vi "UpdateValve.vi"(8 "error in (no error)":errorcluster, 11 "Pump_1AI_1DO_2DI in":refnum<class "Valve_2DO_2DI.lvclass">) -> (0 "error out":errorcluster, 3 "Pump_1AI_1DO_2DI out":refnum<class "Valve_2DO_2DI.lvclass">)   [LabVIEW 2019, in "Valve_2DO_2DI.lvclass"]
uses:
  Valve_2DO_2DI.lvclass
  C:/Users/H4001/Documents/GitHub/H4000/src/Device_class/Device.lvclass
  Device_class/Device.lvclass/Device.ctl
  Valve_2DO_2DI.lvclass/Valve_2DO_2DI.ctl
  DA_class/DA.lvclass/DA.ctl
  Proccess_class/Proccess.lvclass/Proccess.ctl
  FPGA/TypeDef/valveState.ctl
  subvis/bool_change.vi
  DA_class/private/write_to_db.vi
  Proccess_class/GetNames.vi
  Proccess_class/GetLogger.vi
  DA_class/DA.lvclass
  C:/Users/H4001/Documents/GitHub/H4000/src/Proccess_class/Proccess.lvclass
  Logger_class/WriteEvent.vi
  FPGA_API_class/FPGA API.lvclass
  Device_class/Device.lvclass
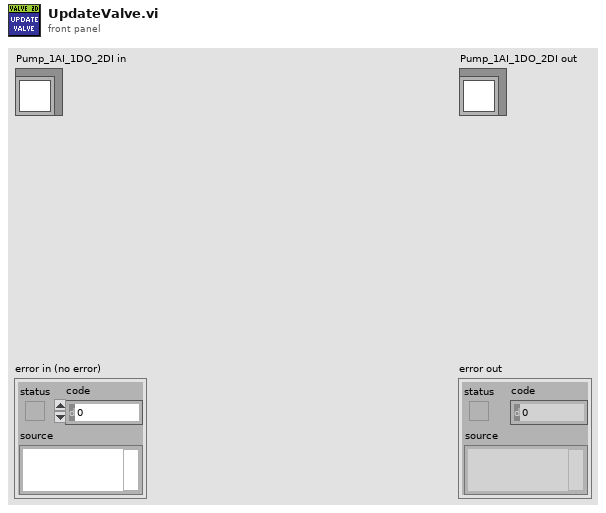
[diagram p1: front panel]
types:
  T1 = typedef "valveState.ctl" = enum16{"Unknown", "Closed", "Opening", "Opened", "Closing"}
  T2 = typedef "DI index.ctl" = u8
  T3 = typedef "DO index.ctl" = u8
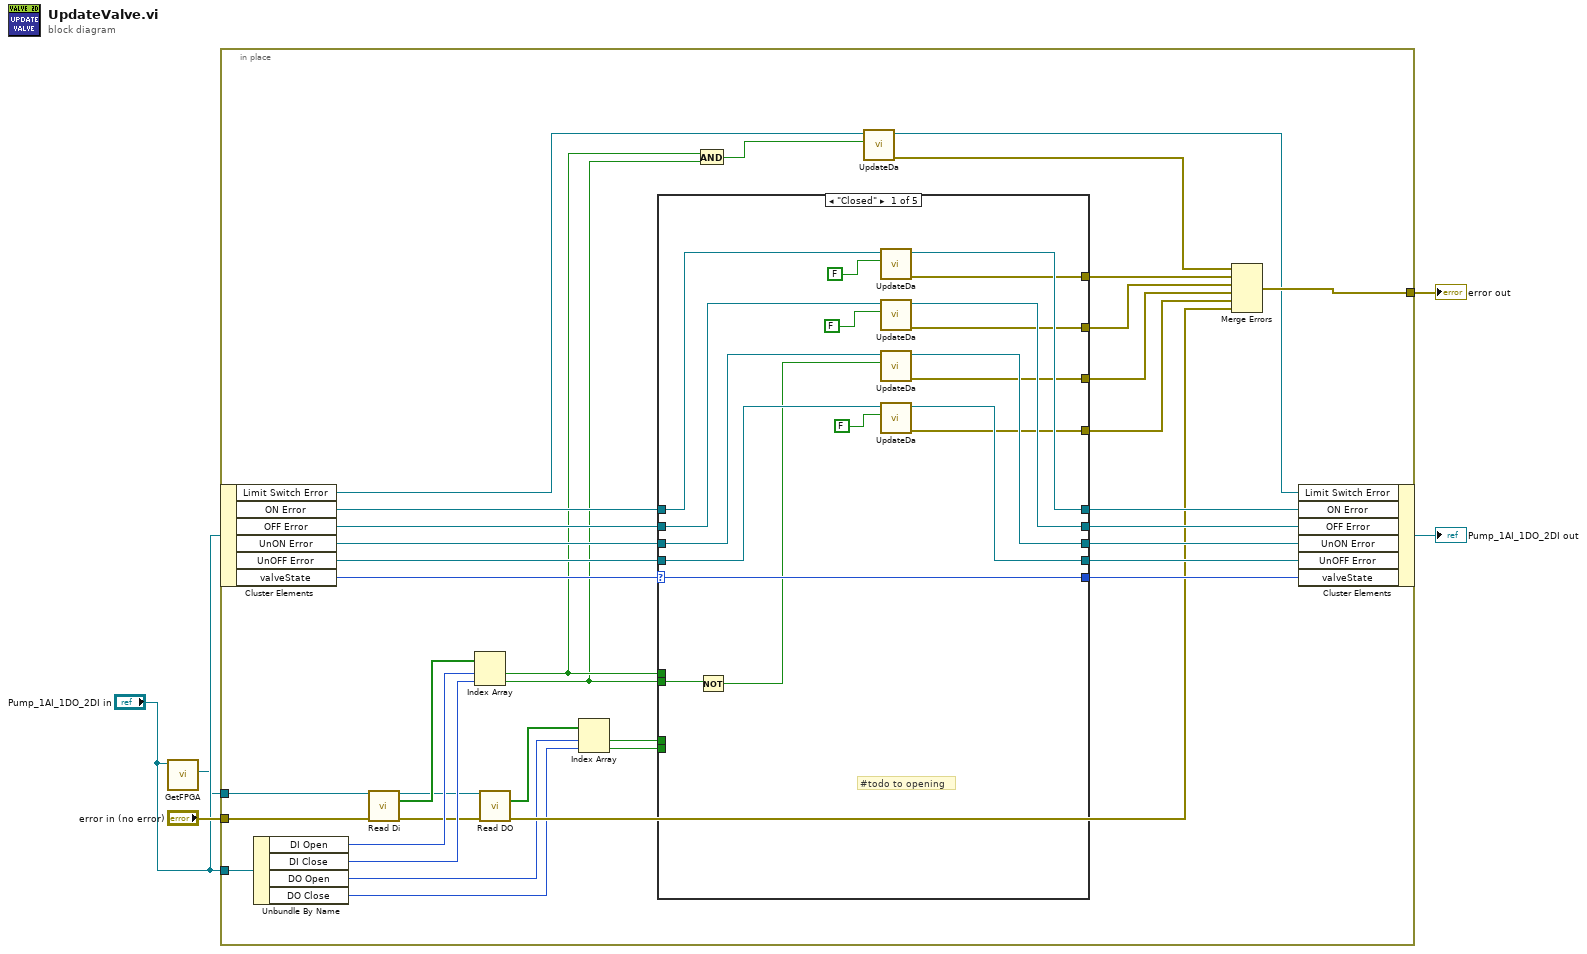
[diagram p0: block diagram]
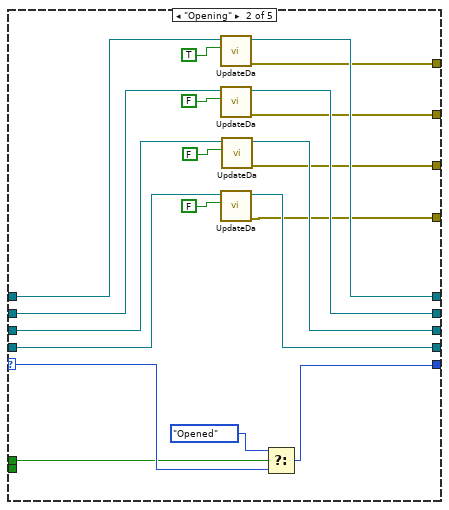
[diagram p2: hidden frame]
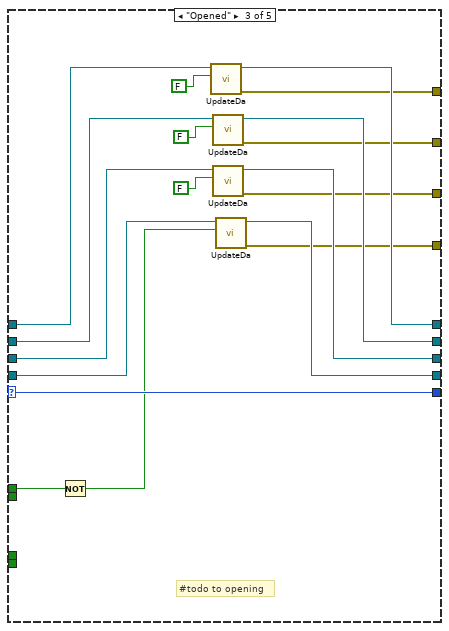
[diagram p3: hidden frame]
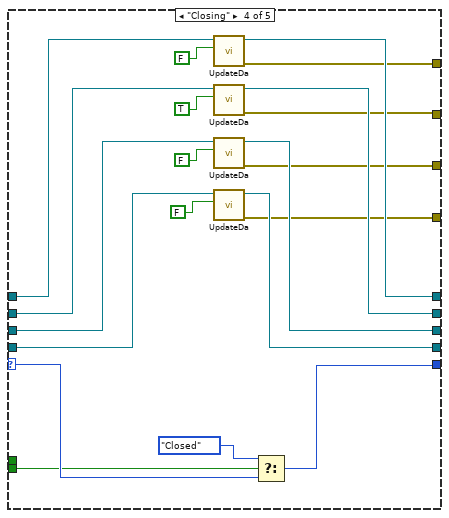
[diagram p4: hidden frame]
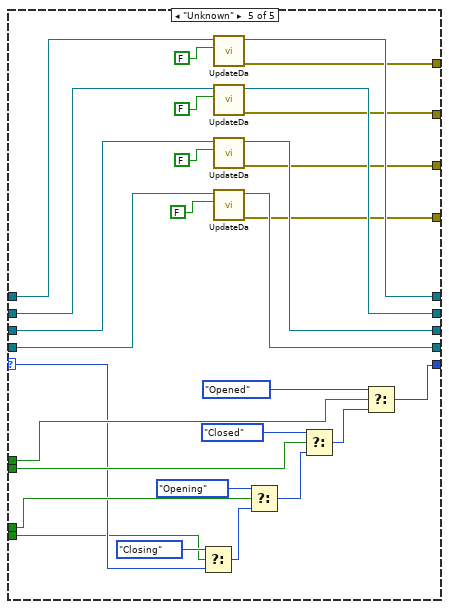
[diagram p5: hidden frame]
diagram:
  n1 = call "GetFPGA.vi"("Device in"="Pump_1AI_1DO_2DI in") -> ("FPGA API.lvclass"=w1:refnum<class "FPGA API.lvclass">)  [unwired: 10 in]
  n2 = in-place {
    in-place-border: "error in (no error)" -> [w21]
    in-place-border: [w26] -> w4
    in-place-border: "Pump_1AI_1DO_2DI in" -> [w25]
    in-place-border: w1 -> [w14]
    n3 = in-place-cluster #1("Pump_1AI_1DO_2DI in") -> ("Limit Switch Error"=w20:refnum<class "DA.lvclass">, "ON Error"=w36:refnum<class "DA.lvclass">, "OFF Error"=w34:refnum<class "DA.lvclass">, "UnON Error"=w38:refnum<class "DA.lvclass">, "UnOFF Error"=w32:refnum<class "DA.lvclass">, "valveState"=w40:T1)
    n4 = Unbundle By Name(w25) -> ("DI Open"=w23:T2, "DI Close"=w22:T2, "DO Open"=w9:T3, "DO Close"=w8:T3)
    n5 = call "Read Di.vi"("FPGA API in"=w14, "error in (no error)"=w21) -> ("FPGA API out"=w13:refnum<class "FPGA API.lvclass">, "DIs"=w24:bool[], "error out"=w12:errorcluster)  [unwired: 11 in]
    n6 = Index Array(array=w24, index #1=w23, index #2=w22) -> (element #1=w17:bool, element #2=w16:bool)
    n7 = call "Read DO.vi"("FPGA API in"=w13, "error in (no error)"=w12) -> ("Ds"=w10:bool[], "error out"=w11:errorcluster)  [unwired: 11 in, 1 out]
    n8 = Index Array(array=w10, index #1=w9, index #2=w8) -> (element #1=w7:bool, element #2=w6:bool)
    n9 = case shown="\"Closed\"" w40 {
      selector: w40 -> [w58 w78 w96 w116 w118]
      tunnel: [w58 w77 w96 w115 w122] -> w39
      tunnel: w38 -> [w57 w68 w88 w106 w137]
      tunnel: [w53 w75 w93 w112 w143] -> w37
      tunnel: w36 -> [w54 w76 w94 w113 w144]
      tunnel: [w50 w69 w89 w109 w140] -> w35
      tunnel: w34 -> [w51 w70 w90 w110 w141]
      tunnel: [w47 w65 w85 w104 w135] -> w33
      tunnel: w32 -> [w48 w66 w86 w105 w136]
      tunnel: [w56 w67 w87 w103 w134] -> w31
      tunnel: [w46 w61 w80 w99 w130] -> w27
      tunnel: [w45 w62 w81 w100 w131] -> w28
      tunnel: [w44 w63 w82 w102 w133] -> w29
      tunnel: [w43 w64 w83 w101 w132] -> w30
      tunnel: w17 -> [_ w60 w79 _ w126]
      tunnel: w16 -> [w42 _ _ w97 w128]
      tunnel: w7 -> [_ _ _ _ w123]
      tunnel: w6 -> [_ _ _ _ w117]
      frame "Closed" {
        # "#todo to opening"
        n10 = Not(x=w42) -> (.not. x?=w41:bool)
        n11 = call "UpdateDa.vi"("RAW"=FALSE, "Sig_DA in"=w54) -> ("error out"=w43:errorcluster, "Sig_DA out"=w53:refnum<class "DA.lvclass">)  [unwired: 7 in, 1 out]
        n12 = call "UpdateDa.vi"("RAW"=FALSE, "Sig_DA in"=w51) -> ("error out"=w44:errorcluster, "Sig_DA out"=w50:refnum<class "DA.lvclass">)  [unwired: 7 in, 1 out]
        n13 = call "UpdateDa.vi"("RAW"=w41, "Sig_DA in"=w57) -> ("error out"=w45:errorcluster, "Sig_DA out"=w56:refnum<class "DA.lvclass">)  [unwired: 7 in, 1 out]
        n14 = call "UpdateDa.vi"("RAW"=FALSE, "Sig_DA in"=w48) -> ("error out"=w46:errorcluster, "Sig_DA out"=w47:refnum<class "DA.lvclass">)  [unwired: 7 in, 1 out]
      }
      frame "Opening" {
        n15 = call "UpdateDa.vi"("RAW"=TRUE, "Sig_DA in"=w76) -> ("error out"=w64:errorcluster, "Sig_DA out"=w75:refnum<class "DA.lvclass">)  [unwired: 7 in, 1 out]
        n16 = call "UpdateDa.vi"("RAW"=FALSE, "Sig_DA in"=w70) -> ("error out"=w63:errorcluster, "Sig_DA out"=w69:refnum<class "DA.lvclass">)  [unwired: 7 in, 1 out]
        n17 = call "UpdateDa.vi"("RAW"=FALSE, "Sig_DA in"=w66) -> ("error out"=w61:errorcluster, "Sig_DA out"=w65:refnum<class "DA.lvclass">)  [unwired: 7 in, 1 out]
        n18 = call "UpdateDa.vi"("RAW"=FALSE, "Sig_DA in"=w68) -> ("error out"=w62:errorcluster, "Sig_DA out"=w67:refnum<class "DA.lvclass">)  [unwired: 7 in, 1 out]
        n19 = Select(t=valveState."Opened" ("valveState"), s=w60, f=w78) -> (s? t:f=w77:T1)
      }
      frame "Opened" {
        # "#todo to opening"
        n20 = Not(x=w79) -> (.not. x?=w84:bool)
        n21 = call "UpdateDa.vi"("RAW"=FALSE, "Sig_DA in"=w94) -> ("error out"=w83:errorcluster, "Sig_DA out"=w93:refnum<class "DA.lvclass">)  [unwired: 7 in, 1 out]
        n22 = call "UpdateDa.vi"("RAW"=FALSE, "Sig_DA in"=w90) -> ("error out"=w82:errorcluster, "Sig_DA out"=w89:refnum<class "DA.lvclass">)  [unwired: 7 in, 1 out]
        n23 = call "UpdateDa.vi"("RAW"=FALSE, "Sig_DA in"=w88) -> ("error out"=w81:errorcluster, "Sig_DA out"=w87:refnum<class "DA.lvclass">)  [unwired: 7 in, 1 out]
        n24 = call "UpdateDa.vi"("RAW"=w84, "Sig_DA in"=w86) -> ("error out"=w80:errorcluster, "Sig_DA out"=w85:refnum<class "DA.lvclass">)  [unwired: 7 in, 1 out]
      }
      frame "Closing" {
        n25 = call "UpdateDa.vi"("RAW"=FALSE, "Sig_DA in"=w113) -> ("error out"=w101:errorcluster, "Sig_DA out"=w112:refnum<class "DA.lvclass">)  [unwired: 7 in, 1 out]
        n26 = call "UpdateDa.vi"("RAW"=TRUE, "Sig_DA in"=w110) -> ("error out"=w102:errorcluster, "Sig_DA out"=w109:refnum<class "DA.lvclass">)  [unwired: 7 in, 1 out]
        n27 = call "UpdateDa.vi"("RAW"=FALSE, "Sig_DA in"=w106) -> ("error out"=w100:errorcluster, "Sig_DA out"=w103:refnum<class "DA.lvclass">)  [unwired: 7 in, 1 out]
        n28 = call "UpdateDa.vi"("RAW"=FALSE, "Sig_DA in"=w105) -> ("error out"=w99:errorcluster, "Sig_DA out"=w104:refnum<class "DA.lvclass">)  [unwired: 7 in, 1 out]
        n29 = Select(t=valveState."Closed", s=w97, f=w116) -> (s? t:f=w115:T1)
      }
      frame "Unknown" {
        n30 = Select(t=valveState."Closing", s=w117, f=w118) -> (s? t:f=w119:T1)
        n31 = call "UpdateDa.vi"("RAW"=FALSE, "Sig_DA in"=w144) -> ("error out"=w132:errorcluster, "Sig_DA out"=w143:refnum<class "DA.lvclass">)  [unwired: 7 in, 1 out]
        n32 = call "UpdateDa.vi"("RAW"=FALSE, "Sig_DA in"=w141) -> ("error out"=w133:errorcluster, "Sig_DA out"=w140:refnum<class "DA.lvclass">)  [unwired: 7 in, 1 out]
        n33 = call "UpdateDa.vi"("RAW"=FALSE, "Sig_DA in"=w137) -> ("error out"=w131:errorcluster, "Sig_DA out"=w134:refnum<class "DA.lvclass">)  [unwired: 7 in, 1 out]
        n34 = call "UpdateDa.vi"("RAW"=FALSE, "Sig_DA in"=w136) -> ("error out"=w130:errorcluster, "Sig_DA out"=w135:refnum<class "DA.lvclass">)  [unwired: 7 in, 1 out]
        n35 = Select(t=valveState."Opening", s=w123, f=w119) -> (s? t:f=w121:T1)
        n36 = Select(t=valveState."Closed", s=w128, f=w121) -> (s? t:f=w125:T1)
        n37 = Select(t=valveState."Opened", s=w126, f=w125) -> (s? t:f=w122:T1)
      }
    }
    n38 = And(x=w17, y=w16) -> (x .and. y?=w15:bool)
    n39 = call "UpdateDa.vi"("RAW"=w15, "Sig_DA in"=w20) -> ("error out"=w18:errorcluster, "Sig_DA out"=w19:refnum<class "DA.lvclass">)  [unwired: 7 in, 1 out]
    n40 = Merge Errors(w18, w30, w29, w28, w27, w11) -> (w26:errorcluster)
    n41 = in-place-cluster #1("Limit Switch Error"=w19, "ON Error"=w37, "OFF Error"=w35, "UnON Error"=w31, "UnOFF Error"=w33, "valveState"=w39) -> (→"Pump_1AI_1DO_2DI out":refnum<class "Valve_2DO_2DI.lvclass">)
  }
  "error out" <- w4
